vi "Page_Info_Validate_BuildSpec_Name.vi"(8 "error in (no error)":errorcluster, 10 "BuildSpec name":string, 11 "AB_Build in":refnum<class "AB_Build.lvclass">) -> (0 "error out":errorcluster, 1 "hasInvalidCharacters":bool, 3 "AB_Build out":refnum<class "AB_Build.lvclass">, 5 "message":string)   [LabVIEW 2020, in "AB_Build.lvclass"]
uses:
  <vilib>/AppBuilder/AB_Classes/Build/AB_Build.lvclass
  <resource>/Framework/Providers/Common/provcom_StringGlobals.vi
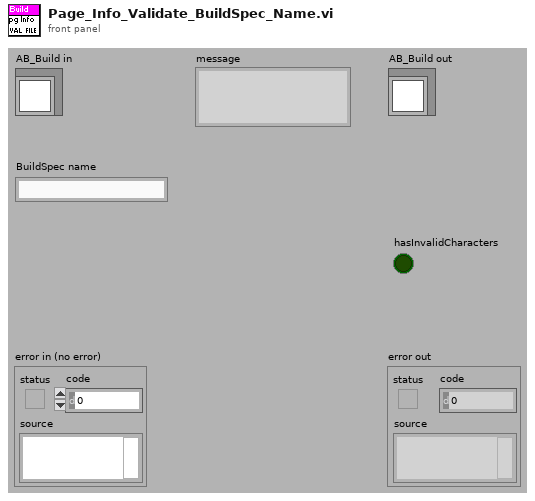
[diagram p1: front panel]
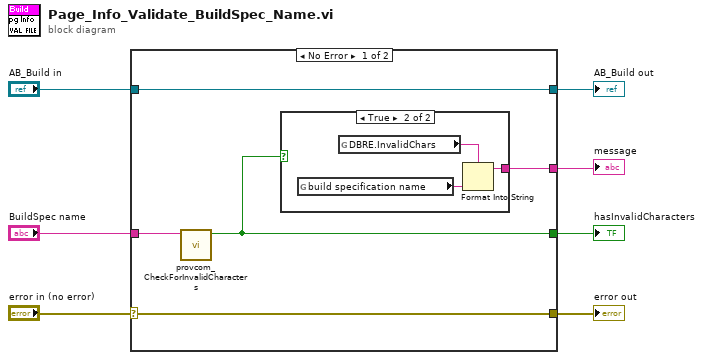
[diagram p0: block diagram]
diagram:
  n1 = case shown="No Error" "error in (no error)" {
    selector: "error in (no error)" -> [w11 w17]
    tunnel: [w11 w17] -> w6
    tunnel: [w12 w16] -> w4
    tunnel: "AB_Build in" -> [w12 w16]
    tunnel: "BuildSpec name" -> [w10 _]
    tunnel: [w8 _] -> w2
    tunnel: [w9 _] -> w1
    frame No Error {
      n2 = call <resource>:"provcom_CheckForInvalidCharacters.vi"("NewString"=w10) -> ("HasInvalidCharacters"=w8:bool)  [unwired: 2 in, 8 out]
      n3 = case shown="True" w8 {
        tunnel: [_ w13] -> w9
        frame False {
        }
        frame True {
          n4 = global read "provcom_StringGlobals.vi" "build specification name"() -> (w14:string)
          n5 = global read "provcom_StringGlobals.vi" "DBRE.InvalidChars"() -> (w15:string)
          n6 = Format Into String(format string=w15, w14) -> (resulting string=w13:string)  [unwired: 2 in, 1 out]
        }
      }
    }
    frame Error {
    }
  }
  "error out" <- w6
  "AB_Build out" <- w4
  "message" <- w1
  "hasInvalidCharacters" <- w2
